vi "search string list.vi"(10 "string to locate":string, 11 "sorted strings":string[](array[string])) -> (3 "index":i32)   [LabVIEW 2013, in "tag bus.lvlib" / "binary search.lvlib"]
doc: "performs a binary search on the input array. It <b>assumes</b> that the input list is sorted and the string to search for is not empty. If the string is not found, -1 is returned."
uses:
  binary search.lvlib
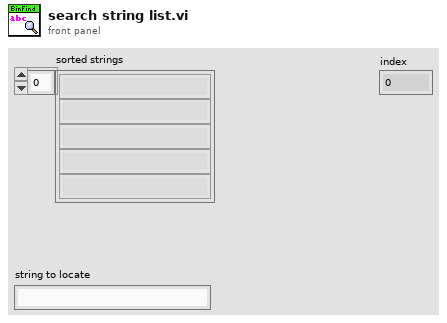
[diagram p1: front panel]
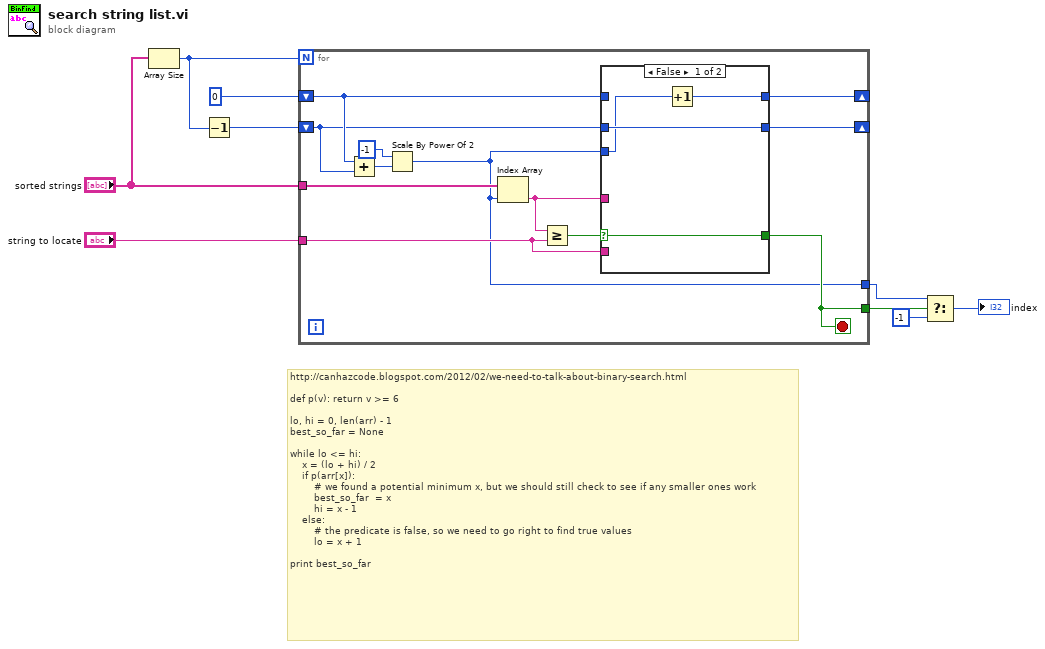
[diagram p0: block diagram]
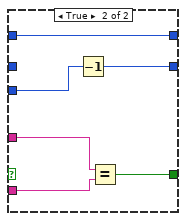
[diagram p2: hidden frame]
diagram:
  # "http://canhazcode.blogspot.com/2012/02/we-need-to-talk-about-binary-search.html\n\ndef p(v): return v >= 6\n \nlo, hi = 0, len(arr) - 1\nbest_so_far = None\n \nwhile lo <= hi:\n    x = (lo + hi) / 2\n    if p(arr[x]):\n        # we found a potential minimum x, but we should still check to see if any smaller ones work\n        best_so_far  = x\n        hi = x - 1\n    else:\n        # the predicate is false, so we need to go right to find true values\n        lo = x + 1\n \nprint best_so_far"
  n1 = Array Size(array="sorted strings") -> (size(s)=w9:i32)
  n2 = Decrement(x=w9) -> (x-1=w8:i32)
  n3 = for {
    N: w9 -> [_]
    shift-right: [w10] -> _
    shift-left: w8 -> [w12]
    shift-right: [w11] -> _
    shift-left: 0 -> [w13]
    tunnel: "sorted strings" -> [w19]
    tunnel: "string to locate" -> [w16]
    tunnel: [w17] -> w4
    tunnel: [w14] -> w3
    stop <- w17 stop-if-true
    n4 = Add(x=w13, y=w12) -> (x+y=w21:i32)
    n5 = Scale By Power Of 2(n=i16 -1, x=w21) -> (x*2^n=w14:i32)
    n6 = Index Array(array=w19, index=w14) -> (element=w15:string)
    n7 = Greater Or Equal?(x=w15, y=w16) -> (x >= y?=w18:bool)
    n8 = case shown="False" w18 {
      selector: w18 -> [w25 _]
      tunnel: [w25 w29] -> w17
      tunnel: w16 -> [_ w31]
      tunnel: w15 -> [_ w30]
      tunnel: w14 -> [w22 w27]
      tunnel: w13 -> [_ w28]
      tunnel: w12 -> [w24 _]
      tunnel: [w23 w28] -> w11
      tunnel: [w24 w26] -> w10
      frame False {
        n9 = Increment(x=w22) -> (x+1=w23:i32)
      }
      frame True {
        n10 = Decrement(x=w27) -> (x-1=w26:i32)
        n11 = Equal?(x=w30, y=w31) -> (x = y?=w29:bool)
      }
    }
  }
  n12 = Select(t=w3, s=w4, f=-1) -> (s? t:f=→"index":i32)
